vi "JKI Open URL In Browser__jki_lib_communication -- VI Tester.vi"(4 "error in (no error)":errorcluster, 5 "run minimized? (F)":bool, 7 "url":string) -> (0 "error out":errorcluster, 3 "duplicate url":string)   [LabVIEW 2011]
doc: "Opens URL in default browser"
uses:
  <vilib>/Platform/browser.llb/Open URL in Default Browser (string).vi
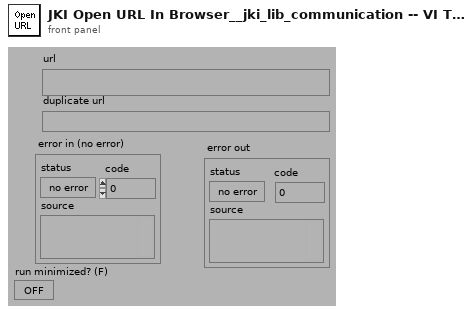
[diagram p1: front panel]
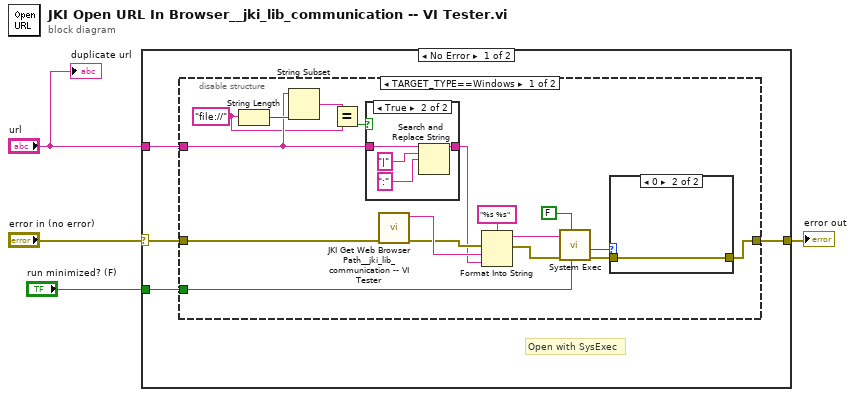
[diagram p0: block diagram]
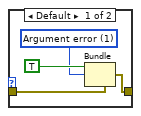
[diagram p3: hidden frame]
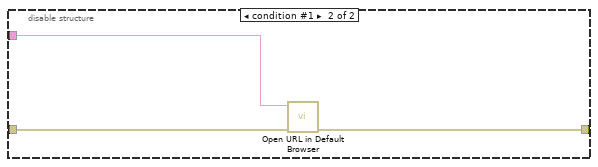
[diagram p4: hidden frame]
diagram:
  n1 = case shown="No Error" "error in (no error)" {
    selector: "error in (no error)" -> [w7 w39]
    tunnel: "url" -> [w8 _]
    tunnel: [w6 w39] -> w4
    tunnel: "run minimized? (F)" -> [w5 _]
    frame No Error {
      # "Open with SysExec"
      n2 = disable-structure shown="TARGET_TYPE==Windows" {
        disable-tunnel: w8 -> [w13 w38]
        disable-tunnel: w7 -> [w23 w37]
        disable-tunnel: [w16 w36] -> w6
        disable-tunnel: w5 -> [w9 _]
        frame condition #0 (active) {
          w11 = "file://" ("search string")
          n3 = String Length(string=w11) -> (length=w14:i32)
          n4 = String Subset(string=w13, length (rest)=w14) -> (substring=w12:string)  [unwired: 1 in]
          n5 = Equal?(x=w12, y=w11) -> (x = y?=w10:bool)
          n6 = case shown="True" w10 {
            tunnel: [w26 w30] -> w15
            tunnel: w13 -> [w26 w27]
            frame False {
            }
            frame True {
              n7 = Search and Replace String(input string=w27, search string="|", replace string=":" ("replace string (\"\")")) -> (result string=w30:string)  [unwired: 5 in, 3 out]
            }
          }
          n8 = call "JKI Get Web Browser Path__jki_lib_communication -- VI Tester.vi"("error in (no error)"=w23) -> ("error out"=w22:errorcluster, "browser command"=w24:string)  [unwired: 5 in]
          n9 = Format Into String(format string="%s %s", error in=w22, w24, w15) -> (resulting string=w18:string, error out=w17:errorcluster)  [unwired: 1 in]
          n10 = call <vilib>:"System Exec.vi"("run minimized? (F)"=w9, "wait until completion? (T)"=FALSE, "error in (no error)"=w17, "command line"=w18) -> ("error out"=w21:errorcluster, "return code"=w20:i32)  [unwired: 4 in, 2 out]
          n11 = case shown="0" w20 {
            tunnel: w21 -> [w34 w35]
            tunnel: [w33 w35] -> w16
            frame Default {
              w31 = 1 items=["No error", "Argument error", "Memory is full", "Out of zone", "End of file", "File already open", "Generic file I/O error", "File not found", "File permission error", "Disk is full", "Duplicate path", "Too many files open", "System feature not enabled", "Resource file not found", "Cannot add resource", "Resource not found", "Image not found", "Image memory error", "Pen does not exist", "Config type invalid", "Config token not found", "Config parse error", "Config memory error", "Bad external code format", "Bad external code offset", "External code not present", "Null window", "Destroy window error", "Null menu", "Print aborted", "Bad print record", "Print driver error", "Windows error during printing", "Memory error during printing", "Print dialog error", "Generic print error", "Invalid device refnum", "Device not found", "Device parameter error", "Device unit error", "Cannot open device", "Device call aborted", "Generic error", "Cancelled by user", "Object ID too low", "Object ID too high", "Object not in heap", "Unknown heap", "Unknown object (invalid DefProc)", "Unknown object (DefProc not in table)", "Message out of range", "Invalid (null) method", "Unknown message", "Manager call not supported", "Bad address", "Network operation in progress", "Network operation timed out", "Connection is busy", "Network attribute not supported", "Network error", "Address in use", "System out of memory", "Connection aborted", "Connection refused", "Not connected", "Already connected", "Connection closed", "Initialization error (interapplication manager)", "Bad occurrence", "Wait on unbound occurrence handler", "Occurrence queue overflow", "Datalog type conflict", "Unused", "Unrecognized type (interapplication manager)", "Memory corrupt", "Failed to make temporary DLL", "Old CIN version", "Drag socket not found", "Failed to load drop-object", "Failed to register OLE object", "Failed to release OLE object", "Format specifier type mismatch", "Unknown format specifier", "Too few format specifiers", "Too many format specifiers", "Scan failed", "Newer CIN version", "Error converting to variant", "Runtime menu error", "Password tampered", "Variant attribute not found", "Incompatible variant data type", "Event data is not available", "Event Store is not present", "Occurrence is not found", "Event Queue is not created", "Event info is not available", "Refnum passed is NULL", "Error retrieving Class GUID", "Error retrieving CoClass GUID", "Error retrieving TypeLib GUID.", "Bad built application magic bytes.", "Specific driver is different from the specific driver associated with the Logical Name.", "There is no session opened to the class driver.", "Max Error", "MAX - Error with config objects", "MAX - Error loading configuration", "MAX - Group not supported"]
              n12 = Bundle(cluster=w34, "status"=TRUE, "code"=w31) -> (w33:errorcluster)  [unwired: 1 in]
            }
            frame 0 {
            }
          }
        }
        frame condition #1 {
          n13 = call-poly <vilib>:"Open URL in Default Browser.vi"("error in (no error)"=w37, "URL"=w38) -> ("error out"=w36:errorcluster)  [unwired: 4 in, 1 out]
        }
      }
    }
    frame Error {
    }
  }
  "error out" <- w4
  "duplicate url" <- "url"
